vi "ReadB.vi"() -> ()   [LabVIEW 2013]
panel:
  in  "error in (no error)":errorcluster
  out "error out":errorcluster
  out "String 4":string
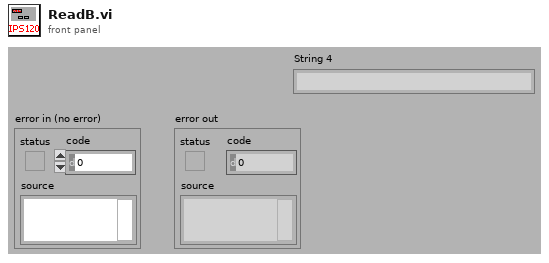
[diagram p1: front panel]
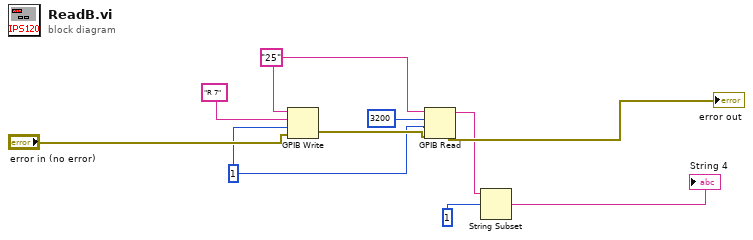
[diagram p0: block diagram]
diagram:
  w4 = 1
  w6 = "25"
  n1 = GPIB Write(0:w6, 1:"R 7", 2:w4, 3:"error in (no error)") -> (6:w10:errorcluster)  [unwired: 1 in, 1 out]
  n2 = GPIB Read(0:w6, 1:3200, 2:w4, 3:w10) -> (5:w3:string, 7:→"error out":errorcluster)  [unwired: 1 in, 1 out]
  n3 = String Subset(string=w3, offset (0)=1) -> (substring=→"String 4":string)  [unwired: 1 in]
